vi "Write Reverse Proxy URI.vi"(8 "error in (no error)":errorcluster, 10 "Reverse Proxy URI":string, 11 "Oauth2 in":refnum<class "Oauth2.lvclass">) -> (0 "error out":errorcluster, 3 "Oauth2 out":refnum<class "Oauth2.lvclass">)   [LabVIEW 2013, in "Oauth2.lvclass"]
uses:
  Oauth2.lvclass
  Oauth2.lvclass/Oauth2.ctl
  OAuthToken/OAuth2 Token Element -- enum.ctl
  <vilib>/LabVIEW Open Source Project/OpenURI/uri/URI.lvclass
  OAuthToken/OAuthAccessToken.lvclass
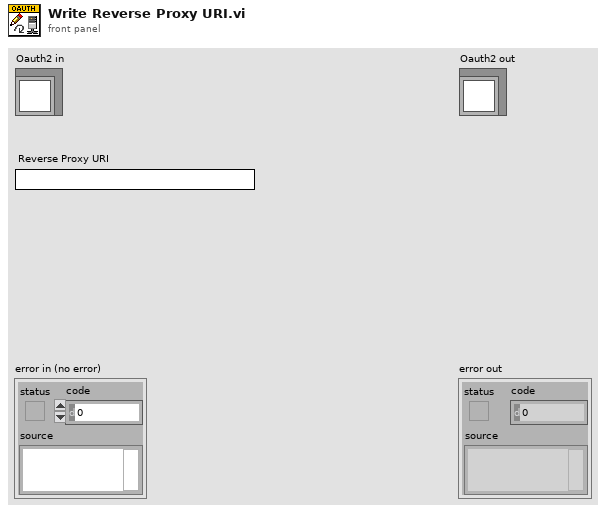
[diagram p1: front panel]
types:
  T1 = typedef "OAuthAccessToken.lvclass/OAuth2 Token Element -- enum.ctl" = enum16{"client_id", "client_secret", "response_type", "scope", "redirect_uri", "error", "error_description", "error_uri", "grant_type", "code", "access_token", "token_type", "expires_in", "username", "password", "refresh_token", "code_challenge", "code_challenge_method", "reverse_proxy_uri", "endpoint element"}
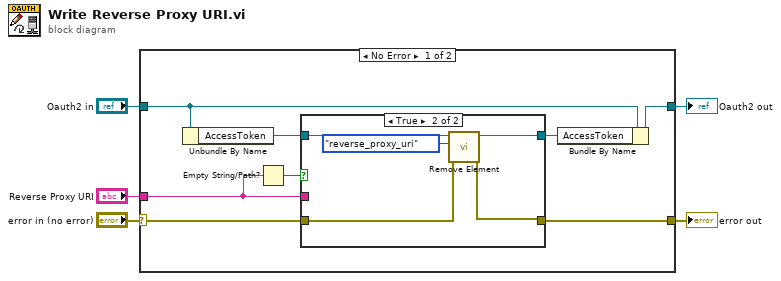
[diagram p0: block diagram]
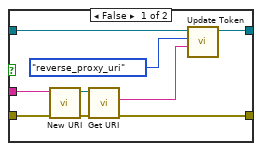
[diagram p2: hidden frame]
diagram:
  n1 = case shown="No Error" "error in (no error)" {
    selector: "error in (no error)" -> [w9 w28]
    tunnel: [w8 w28] -> w4
    tunnel: [w10 w29] -> w2
    tunnel: "Oauth2 in" -> [w11 w29]
    tunnel: "Reverse Proxy URI" -> [w6 _]
    frame No Error {
      n2 = Unbundle By Name(w11) -> ("AccessToken"=w12:refnum<class "OAuthAccessToken.lvclass">)
      n3 = Empty String/Path?(string/path=w6) -> (empty?=w7:bool)
      n4 = case shown="True" w7 {
        tunnel: w6 -> [w22 _]
        tunnel: [w21 w26] -> w13
        tunnel: w12 -> [w20 w27]
        tunnel: w9 -> [w15 w24]
        tunnel: [w14 w23] -> w8
        frame False {
          n5 = call <vilib>:"New URI.vi"("error in (no error)"=w15, "URI"=w22) -> ("error out"=w16:errorcluster, "URI"=w18:refnum<class "URI.lvclass">)  [unwired: 8 in]
          n6 = call <vilib>:"Get URI.vi"("error in (no error)"=w16, "URI in"=w18) -> ("error out"=w14:errorcluster, "URI String"=w17:string)  [unwired: 7 in, 1 out]
          n7 = call "Update Token.vi"("Value"=w17, "Token element"=OAuth2_Token_Element_--_enum."reverse_proxy_uri", "OAuthAccessToken in"=w20) -> ("OAuthAccessToken out"=w21:refnum<class "OAuthAccessToken.lvclass">)  [unwired: 7 in, 1 out]
        }
        frame True {
          n8 = call "Remove Element.vi"("error in (no error)"=w24, "Token element"=OAuth2_Token_Element_--_enum."reverse_proxy_uri", "OAuthAccessToken in"=w27) -> ("error out"=w23:errorcluster, "OAuthAccessToken out"=w26:refnum<class "OAuthAccessToken.lvclass">)  [unwired: 6 in, 1 out]
        }
      }
      n9 = Bundle By Name(cluster=w11, "AccessToken"=w13) -> (w10:refnum<class "Oauth2.lvclass">)
    }
    frame Error {
    }
  }
  "error out" <- w4
  "Oauth2 out" <- w2
